vi "SinewaveSiggen_USRPRx.vi"() -> ()   [LabVIEW 2021]
uses:
  <vilib>/addons/Modulation/Analog/controls/Complex Data Waveform.ctl
  <vilib>/measure/maspectr.llb/Power Spectrum and PSD Export Mode.ctl
  system stop.vi
  <vilib>/measure/matone.llb/Extract Single Tone Information 1 Chan (CDB).vi
  <vilib>/measure/maspectr.llb/FFT Power Spectrum and PSD for 1 Chan (CDB).vi
  <instrlib>/niUSRP/niUSRP Fetch Rx Data (CDB Cluster).vi
  <vilib>/addons/Modulation/niAMT.lvlib
  <vilib>/measure/NI_MAPro.lvlib
panel:
  in  "Tab Control":enum32{"Page 1", "Page 2"}(tab)
  in  "IQ rate":dbl=100000.0 format="%#_6p"
  in  "carrier frequency":dbl=100000.0 format="%#_6p"
  in  "device names Rx":refnum<k15>
  in  "gain Rx":dbl format="%#_6f"
  out "coerced carrier frequency":dbl=100000.0 format="%#_6p"
  out "coerced IQ rate":dbl=100000.0 format="%#_6p"
  out "Power Spectral Density Graph":cluster{"f0":dbl, "df":dbl, "magnitude":dbl[]}(graph)
  in  "number of samples Rx on USRP":i64=100000
  out "detected power":dbl format="%.2p"
  out "detected peak frequency":dbl format="%.2p"
  out "Waveform Graph":dbl[](graph)
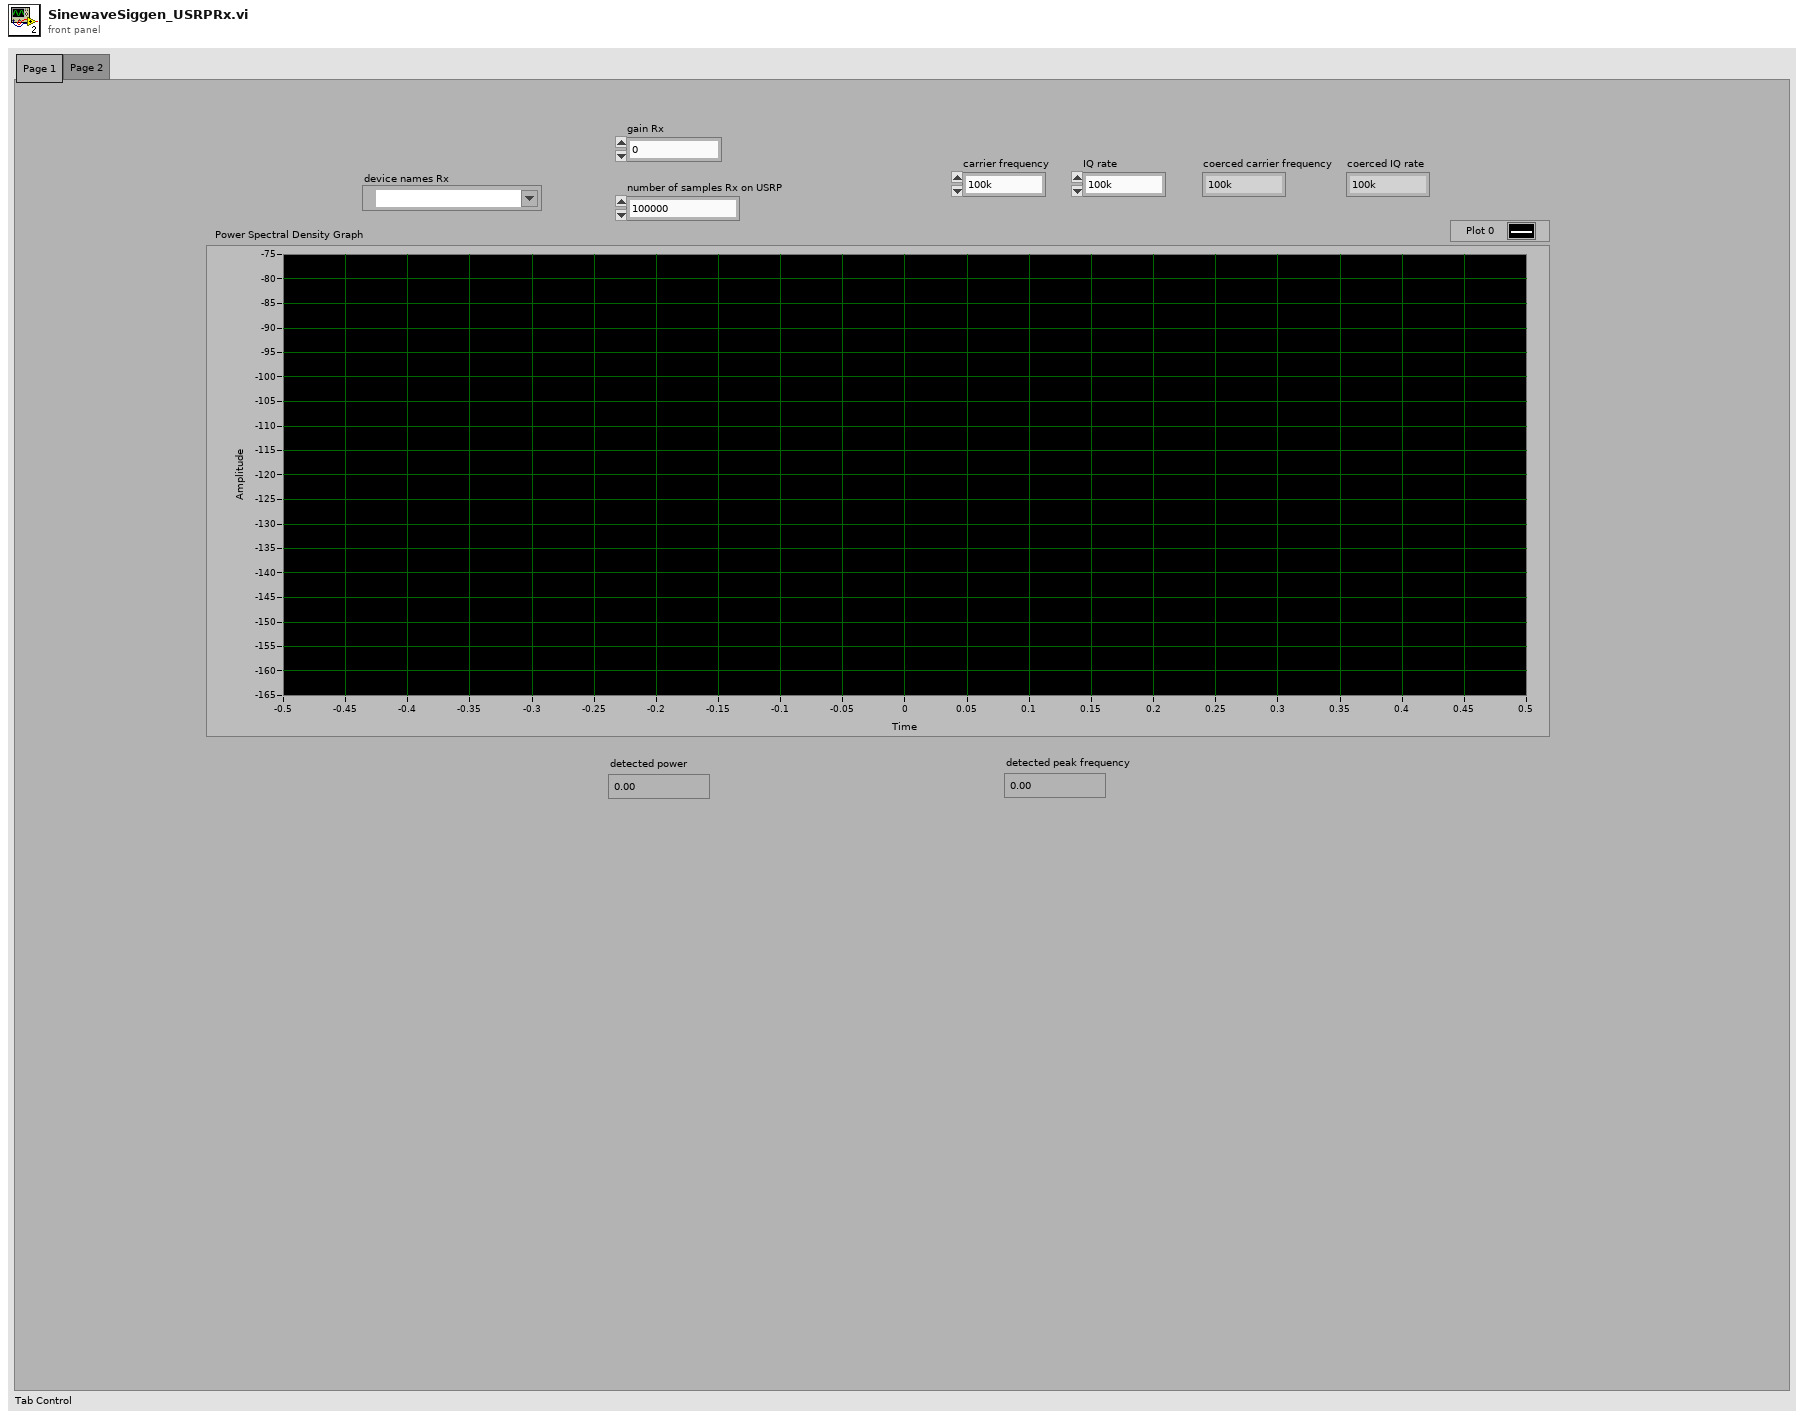
[diagram p1: front panel]
types:
  T1 = typedef "niAMT.lvlib/Complex Data Waveform.ctl" = cluster{"t0":dbl, "dt":dbl, "Y":cdb[]}
  T2 = typedef "NI_MAPro.lvlib/Power Spectrum and PSD Export Mode.ctl" = u16
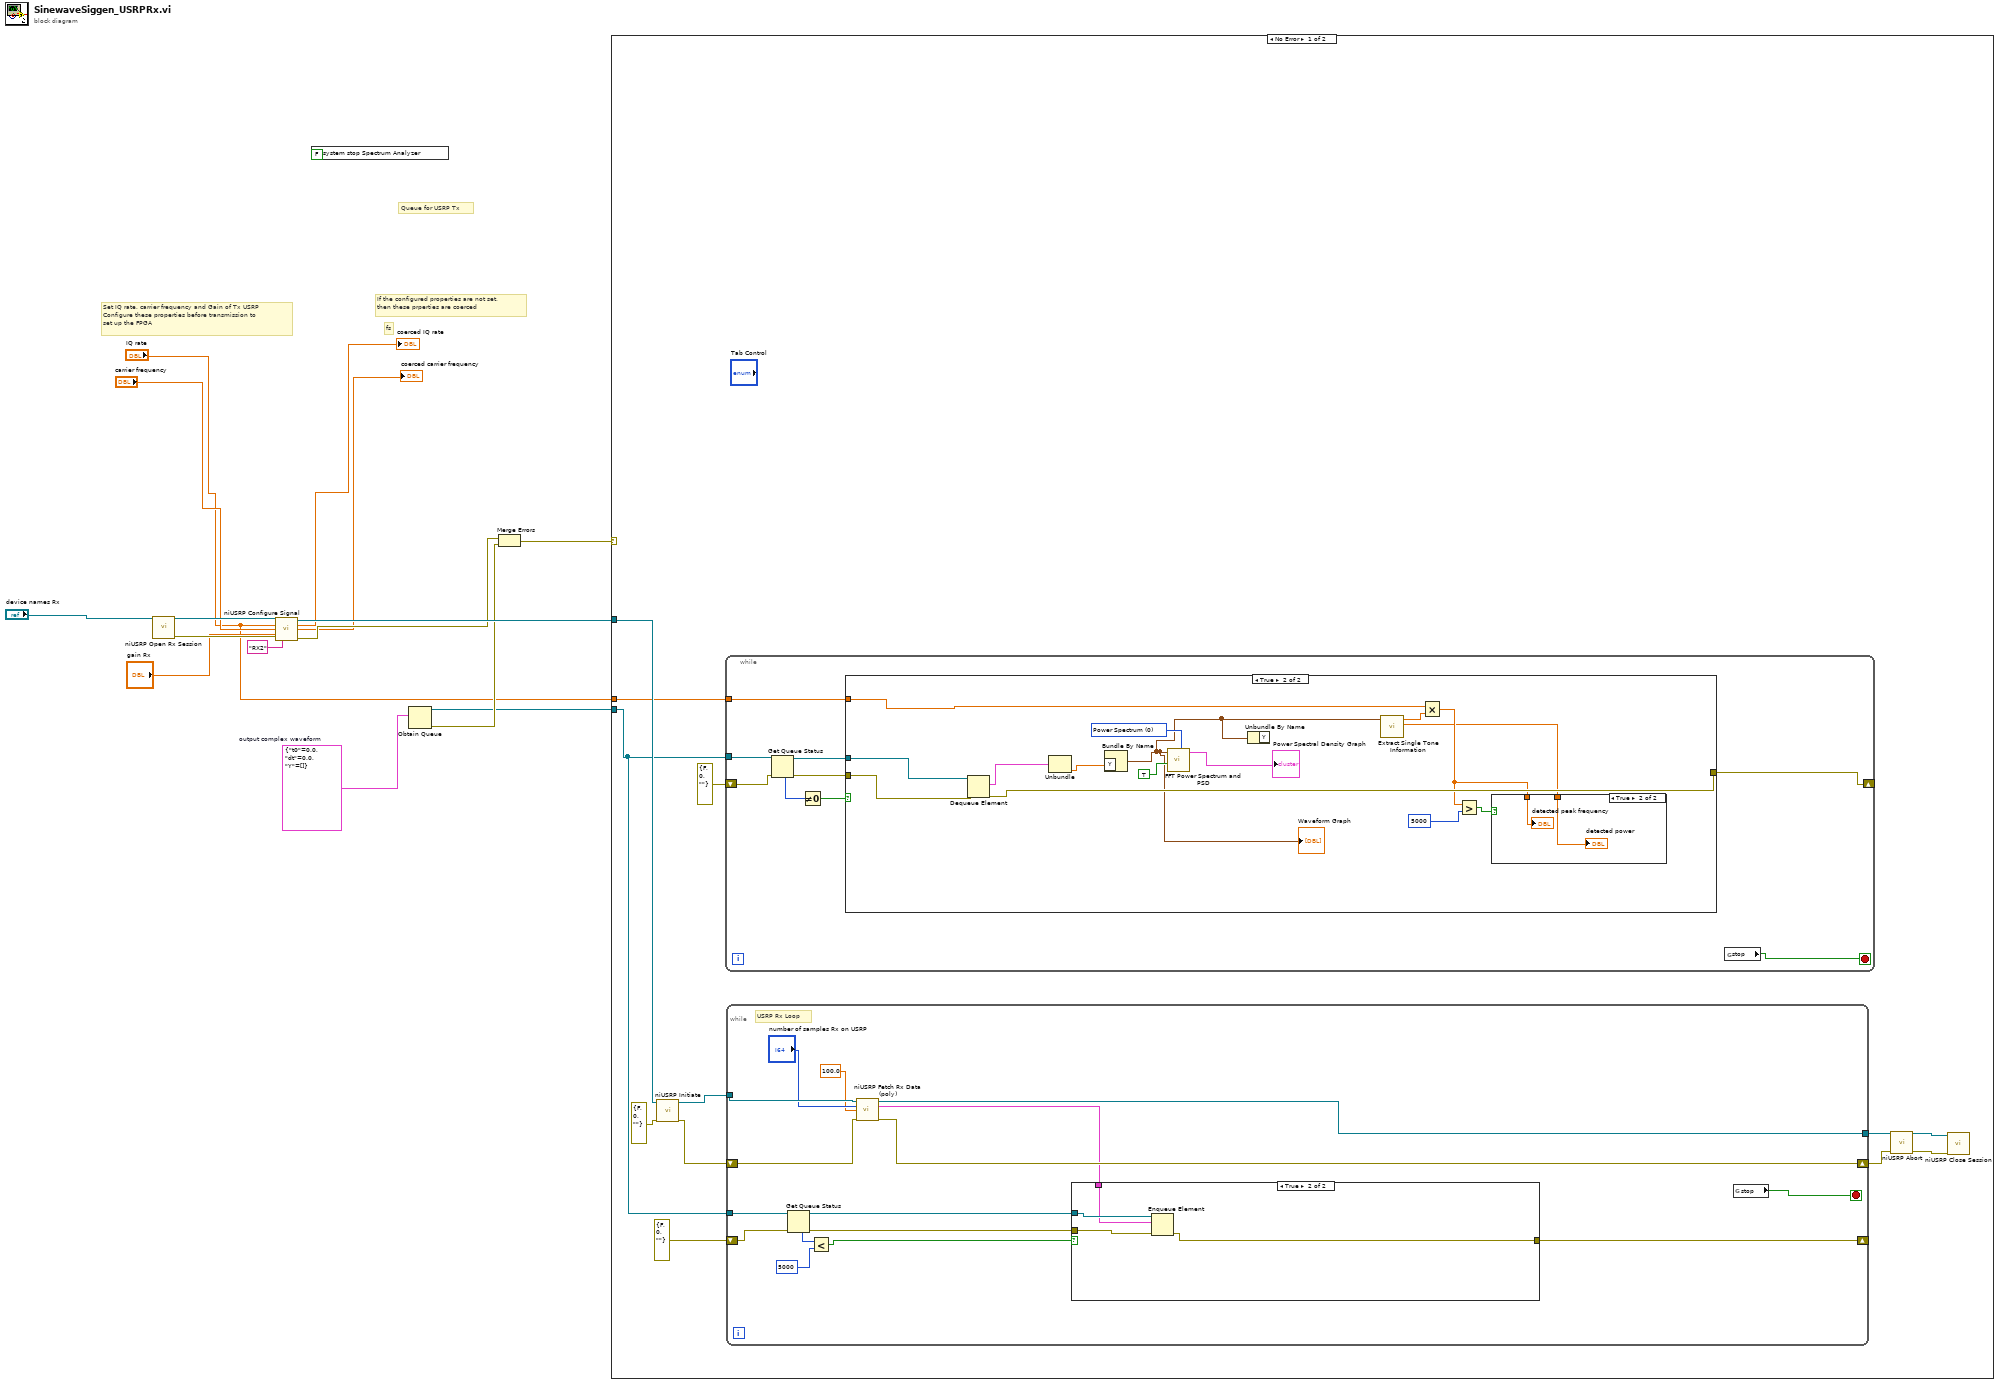
[diagram p0: block diagram]
diagram:
  w9 = T1 {"t0"=0.0, "dt"=0.0, "Y"=[]}  # output complex waveform
  # "fs"
  # "If the configured properties are not set,\nthen these prperties are coerced"
  # "Set IQ rate, carrier frequency and Gain of Tx USRP\nConfigure these properties before transmission to\nset up the FPGA"
  # "Queue for USRP Tx"
  n1 = call <instrlib>:"niUSRP Open Rx Session.vi"("device names"="device names Rx") -> ("session handle out"=w15:refnum<k15>, "error out"=w14:errorcluster)  [unwired: 13 in]
  n2 = call <instrlib>:"niUSRP Configure Signal.vi"("session handle"=w15, "IQ rate"="IQ rate", "carrier frequency"="carrier frequency", "gain"="gain Rx", "error in (no error)"=w14, "active antenna"="RX2") -> ("session handle out"=w10:refnum<k15>, "coerced IQ rate"=→"coerced IQ rate":dbl, "coerced carrier frequency"=→"coerced carrier frequency":dbl, "error out"=w8:errorcluster)  [unwired: 5 in, 1 out]
  n3 = global write "system stop.vi" "system stop Spectrum Analyzer"(FALSE) -> ()
  n4 = Obtain Queue(element data type=w9) -> (queue out=w6:refnum<queue>, error out=w7:errorcluster)  [unwired: 4 in, 1 out]
  n5 = Merge Errors(w8, w7) -> (w12:errorcluster)
  n6 = case shown="No Error" w12 {
    tunnel: w10 -> [w23 _]
    tunnel: w6 -> [w21 _]
    tunnel: "IQ rate" -> [w19 _]
    frame No Error {
      n7 = call <instrlib>:"niUSRP Initiate.vi"("session handle"=w23, "error in (no error)"=errorcluster {"status"=FALSE, "code"=0, "source"=""}) -> ("session handle out"=w18:refnum<k15>, "error out"=w17:errorcluster)  [unwired: 12 in]
      n8 = while {
        tunnel: w21 -> [w37]
        shift-right: [w31] -> _
        shift-left: errorcluster {"status"=FALSE, "code"=0, "source"=""} ("error in (no error)") -> [w36]
        tunnel: w19 -> [w29]
        stop <- w30 stop-if-true
        n9 = Get Queue Status(queue=w37, error in (no error)=w36) -> (queue out=w35:refnum<queue>, error out=w34:errorcluster, # elements in queue=w32:i32)  [unwired: 1 in, 5 out]
        n10 = Not Equal To 0?(x=w32) -> (x != 0?=w33:bool)
        n11 = case shown="True" w33 {
          tunnel: w35 -> [_ w51]
          tunnel: w34 -> [w38 w50]
          tunnel: [w38 w53] -> w31
          tunnel: w29 -> [_ w52]
          frame False {
          }
          frame True {
            w46 = T2 0 items=["Power Spectrum", "Power Spectral Density"] ("export mode")
            n12 = Dequeue Element(queue=w51, error in (no error)=w50) -> (element=w49:T1, error out=w53:errorcluster)  [unwired: 1 in, 2 out]
            n13 = Unbundle(w49) -> ("Y"=w44:cdb[])  [unwired: 2 out]
            n14 = Bundle By Name("Y"=w44) -> (w39:waveform(cdb))  [unwired: 1 in]
            "Waveform Graph" <- w39
            n15 = call-poly <vilib>:"FFT Power Spectrum and PSD.vi"("export mode"=w46, "dB On (F)"=TRUE, "time signal"=w39) -> ("Power Spectrum / PSD"=→"Power Spectral Density Graph":cluster{"f0":dbl, "df":dbl, "magnitude":dbl[]})  [unwired: 5 in, 3 out]
            n16 = Unbundle By Name(w39) -> ()  [unwired: 1 out]
            n17 = call-poly <vilib>:"Extract Single Tone Information.vi"("time signal in"=w39) -> ("detected amplitude"=w40:dbl, "detected frequency"=w45:dbl)  [unwired: 5 in, 4 out]
            n18 = Multiply(x=w52, y=w45) -> (x*y=w41:dbl)
            n19 = Greater?(x=w41, y=5000) -> (0:w42:bool)
            n20 = case shown="True" w42 {
              tunnel: w41 -> [_ w55]
              tunnel: w40 -> [_ w54]
              frame False {
              }
              frame True {
                "detected peak frequency" <- w55
                "detected power" <- w54
              }
            }
          }
        }
        n21 = global read "system stop.vi" "stop"() -> (w30:bool)
      }
      n22 = while {
        tunnel: w18 -> [w71]
        tunnel: [w69] -> w25
        shift-right: [w68] -> w24
        shift-left: w17 -> [w70]
        tunnel: w21 -> [w65]
        shift-right: [w57] -> _
        shift-left: errorcluster {"status"=FALSE, "code"=0, "source"=""} ("error in (no error)") -> [w64]
        stop <- w67 stop-if-true
        # "USRP Rx Loop"
        n23 = Get Queue Status(queue=w65, error in (no error)=w64) -> (queue out=w63:refnum<queue>, error out=w59:errorcluster, # elements in queue=w62:i32)  [unwired: 1 in, 5 out]
        n24 = Less?(x=w62, y=5000) -> (x < y?=w60:bool)
        n25 = call-poly <instrlib>:"niUSRP Fetch Rx Data (poly).vi"("session handle"=w71, "number of samples"="number of samples Rx on USRP", "timeout"=100.0, "error in (no error)"=w70) -> ("session handle out"=w69:refnum<k15>, "data"=w58:cluster{"t0":dbl, "dt":dbl, "Y":cdb[]}, "error out"=w68:errorcluster)  [unwired: 8 in, 1 out]
        n26 = case shown="True" w60 {
          tunnel: w63 -> [_ w76]
          tunnel: w59 -> [w72 w75]
          tunnel: w58 -> [_ w74]
          tunnel: [w72 w73] -> w57
          frame False {
          }
          frame True {
            n27 = Enqueue Element(queue=w76, element=w74, error in (no error)=w75) -> (error out=w73:errorcluster)  [unwired: 1 in, 2 out]
          }
        }
        n28 = global read "system stop.vi" "stop"() -> (w67:bool)
      }
      n29 = call <instrlib>:"niUSRP Abort.vi"("session handle"=w25, "error in (no error)"=w24) -> ("session handle out"=w28:refnum<k15>, "error out"=w27:errorcluster)  [unwired: 12 in]
      n30 = call <instrlib>:"niUSRP Close Session.vi"("session handle"=w28, "error in (no error)"=w27) -> ()  [unwired: 13 in, 1 out]
    }
    frame Error {
    }
  }
